vi "Periodic Tasks.vi"(8 "error in":errorcluster) -> ()   [LabVIEW 2018]
doc: "This VI runs in parallel to other robot code. It can contain as many user-defined periodic loops as you need. These can carry out PID or other sorts of timed response."
uses:
  <vilib>/Utility/config.llb/Read Key (String).vi
  Arm/Implementation/Arm Published Globals.vi
  <vilib>/Rock Robotics/Network Tables/NT Read String.vi
  <vilib>/Utility/config.llb/Write Key (String).vi
  Robot Global Data.vi
  <vilib>/Rock Robotics/SystemInterfaces/DIO/FPGA_DIOChannel.ctl
  <vilib>/ptbypt/NI_PtbyPt.lvlib
  <vilib>/Rock Robotics/WPI/ThirdParty/Phoenix-LabVIEW/Motor Controller/Controls/CTRE_Phoenix_MotorControl_MotionProfileTrajectoryPoint.ctl
  Arm/Arm Positions.ctl
  <vilib>/Utility/config.llb/NI_LVConfig.lvlib
  <vilib>/Rock Robotics/WPI/ThirdParty/Phoenix-LabVIEW/Pigeon IMU/CTRE_PigeonIMU_GetYPR.vi
  <vilib>/Rock Robotics/WPI/ThirdParty/Phoenix-LabVIEW/Motor Controller/Closed Loop/Motion Profile/CTRE_Phoenix_MotorControl_BufferedTrajectoryPointStream_WriteAll.vi
  <vilib>/Utility/file.llb/Read Delimited Spreadsheet (DBL).vi
  <vilib>/Rock Robotics/WPI/Switch/WPI_SwitchOpenCounting.vi
  <vilib>/Rock Robotics/WPI/Switch/WPI_SwitchOpenLimit.vi
panel:
  in  "Read FIle":bool
  out "Switch Pressed":bool
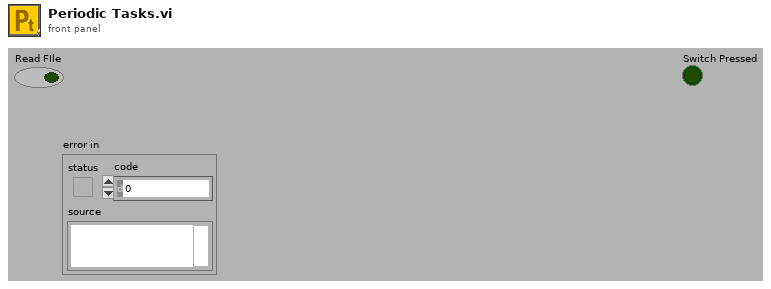
[diagram p1: front panel]
types:
  T1 = typedef "FPGA_DIOChannel.ctl" = enum8{"DIO 0", "DIO 1", "DIO 2", "DIO 3", "DIO 4", "DIO 5", "DIO 6", "DIO 7", "DIO 8", "DIO 9", "DIO MXP 0", "DIO MXP 1", "DIO MXP 2", "DIO MXP 3", "DIO MXP 4", "DIO MXP 5", "DIO MXP 6", "DIO MXP 7", "DIO MXP 8", "DIO MXP 9", "DIO MXP 10", "DIO MXP 11", "DIO MXP 12", "DIO MXP 13", "DIO MXP 14", "DIO MXP 15", "SPI Port CS1", "SPI Port CS2", "SPI Port CS3", "SPI Port MISO", "SPI Port MOSI", "Invalid"}
  T2 = typedef "WPI_JoystickDevRef.ctl" = cluster{"Device":T3}
  T3 = typedef "WPI_JoystickDeviceEnum.ctl" = enum16{"USB 0", "USB 1", "USB 2", "USB 3", "USB 4", "USB 5"}
  T4 = typedef "WPI_SwitchDevRef.ctl" = cluster{"DevStatus":errorcluster, "DIO Channel":T1, "CntIndex":T5, "Normally Closed":bool}
  T5 = typedef "FPGA_CounterCtrSystemIndex.ctl" = enum8{"Ctr 0", "Ctr 1", "Ctr 2", "Ctr 3", "Ctr 4", "Ctr 5", "Ctr 6", "Ctr 7", "Invalid"}
  T6 = typedef "CTRE_Phoenix_MotorControl_MotionProfileTrajectoryPoint.ctl" = cluster{"Position":dbl, "Velocity":dbl, "Arbitrary Feed Forward":dbl, "Auxiliary Position":dbl, "Auxiliary Velocity":dbl, "Auxiliary Arbitrary Feed Forward":dbl, "Profile Slot Select":i32, "Auxiliary Profile Slot Select":i32, "isLastPoint?":bool, "Zero Position?":bool, "durationMs":u32, "Use Aux PID?":bool}
  T7 = typedef "CTRE_Phoenix_MotorControl_BufferedTrajectoryPointStream_DeviceRef.ctl" = cluster{"Handle":u64, "Library Path":path}
  T8 = typedef "Arm Positions.ctl" = enum16{"Home Position", "Safe Position", "Hatch - Ground", "Hatch - Low", "Hatch - Middle", "Hatch - High", "Hatch - High 2", "Cargo - Low", "Cargo - Middle", "Cargo - High", "Cargo - Loading Station", "Hatch - Loading Station", "Cargo - Ground", "Turret - Left", "Turret - Front", "Turret - Right", "Turret - Back", "Climbing - Forward", "Hatch - Middle2"}
  T9 = typedef "CTRE_PigeonIMU_DeviceRef.ctl" = cluster{"DeviceStatus":errorcluster, "Device Number":u8, "Type":T10, "Device ID":u32, "Handle":u64, "UsageFrame":u32, "Library Path":path}
  T10 = typedef "CTRE_PigeonIMU_ConnectionType.ctl" = u32
  T11 = typedef "NI_LVConfig.lvlib/Config Data RefNum.ctl" = refnum<k1>
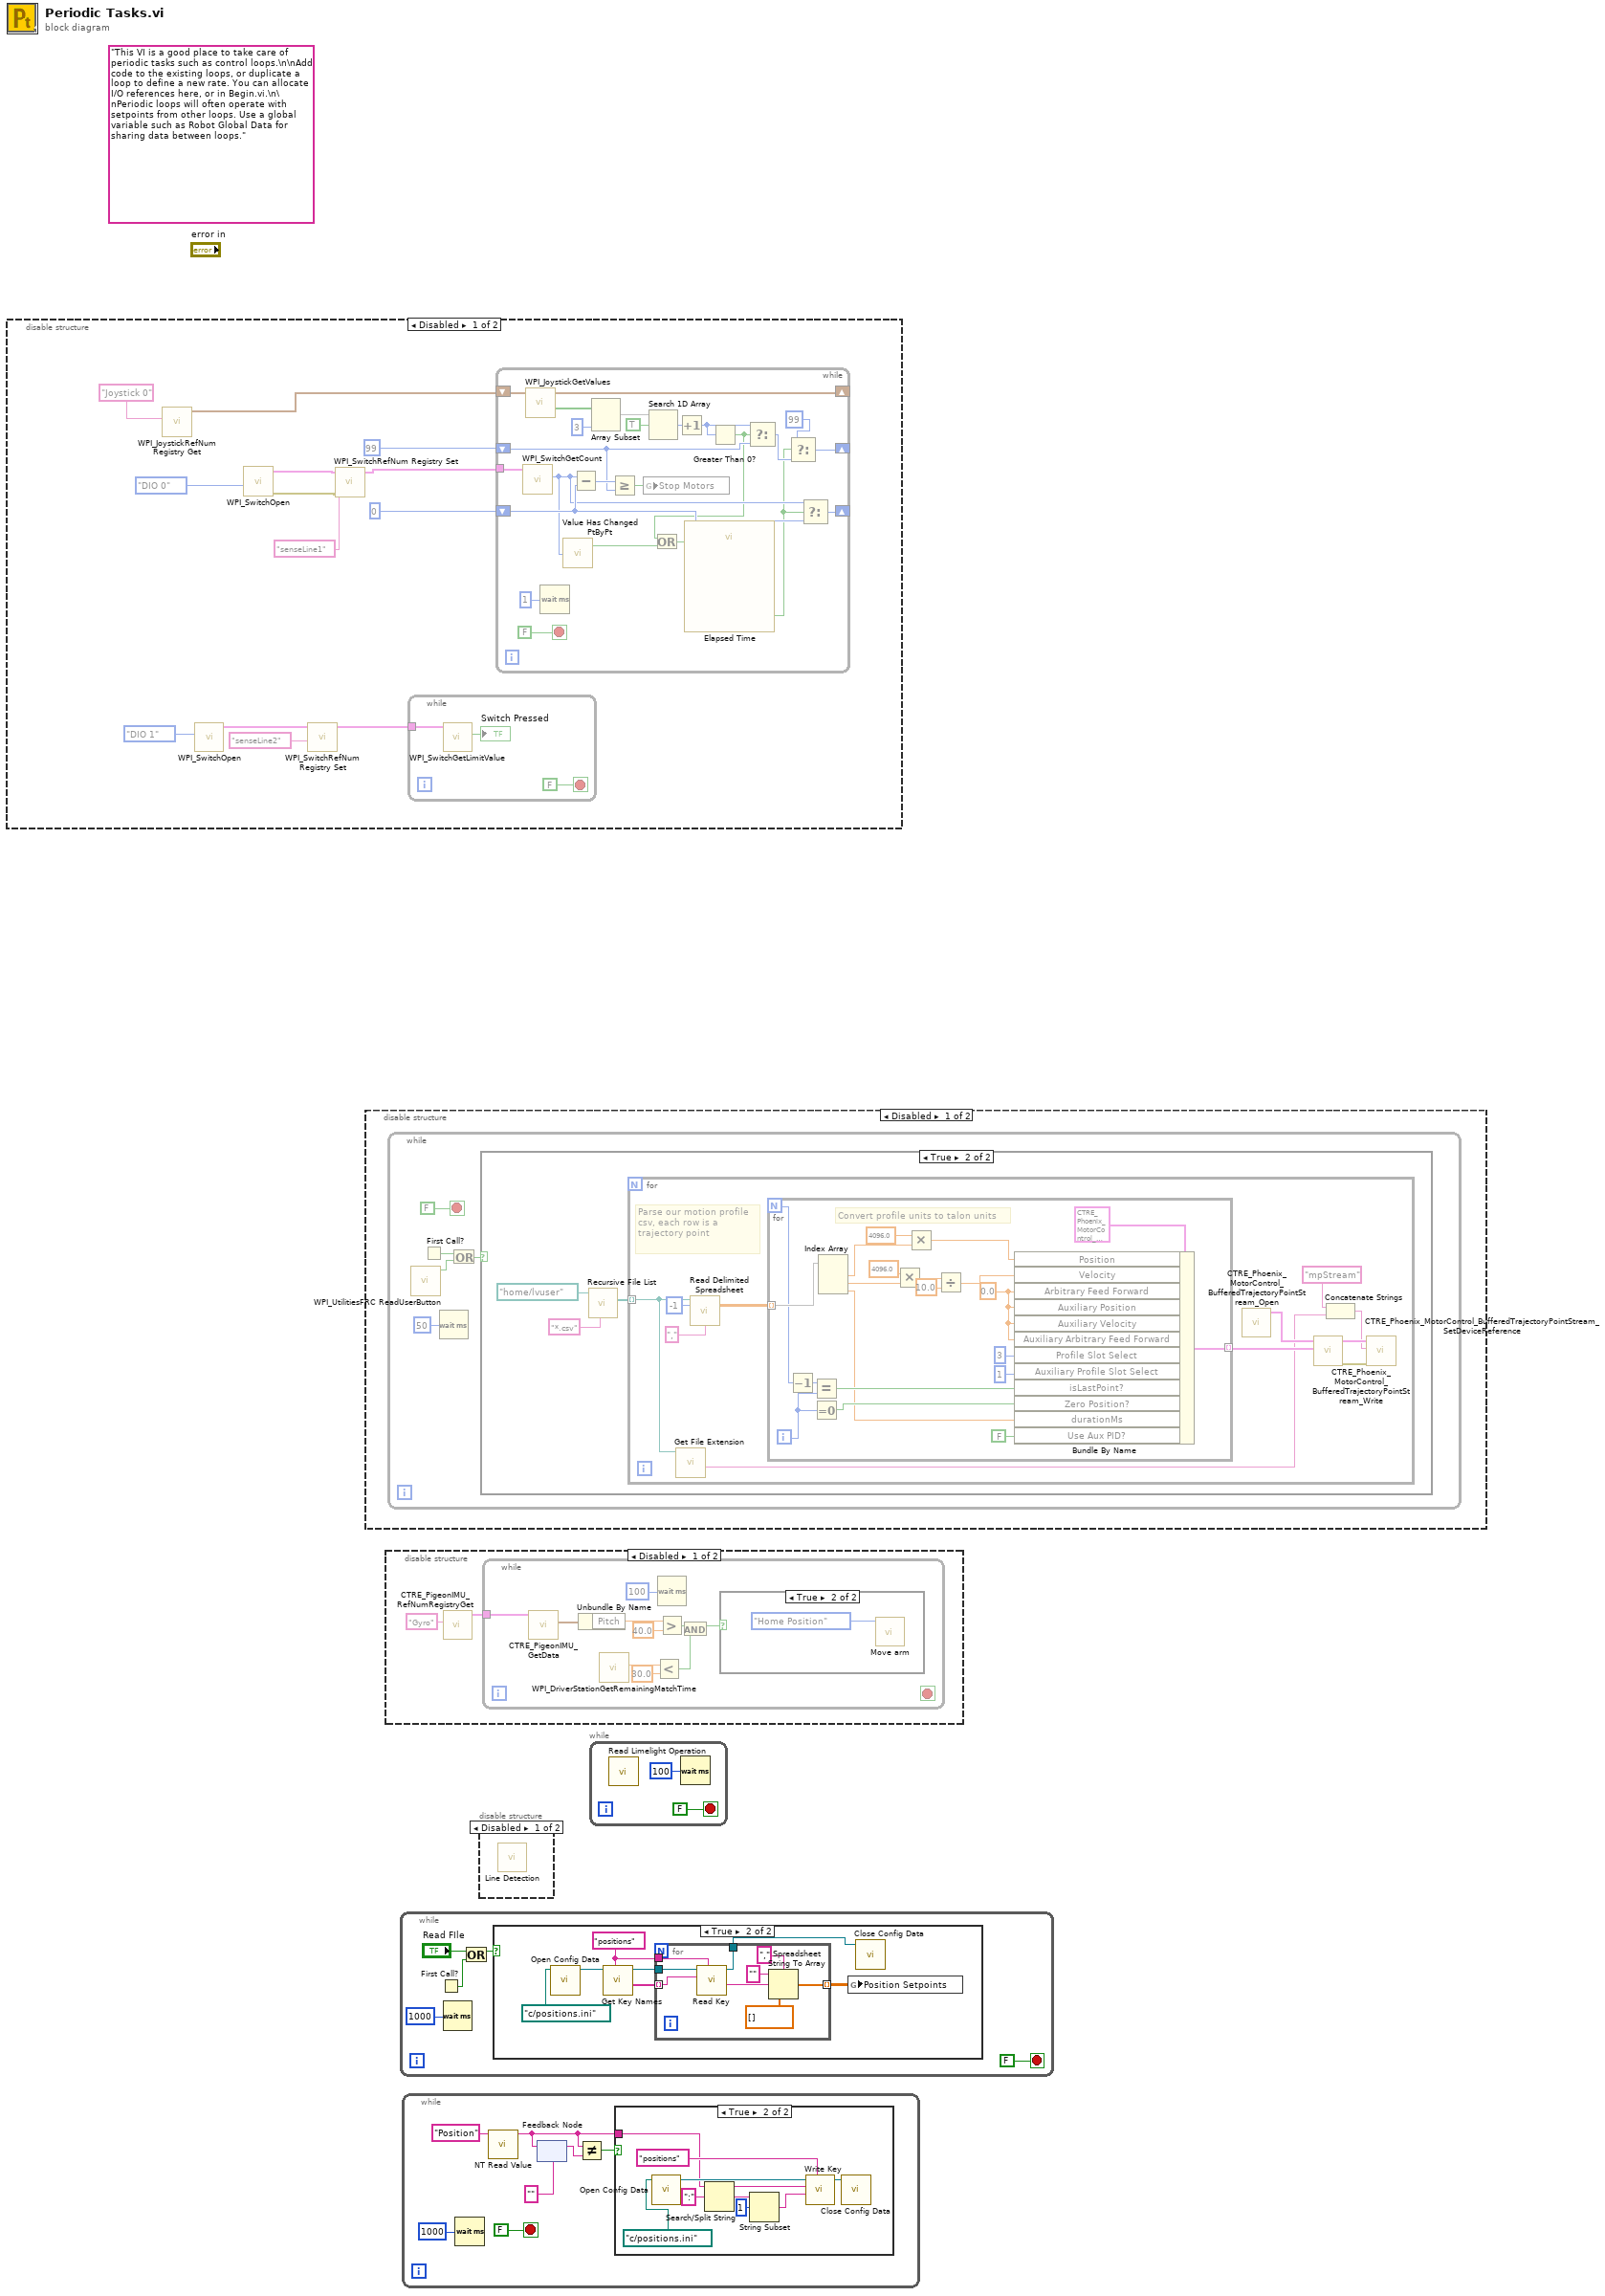
[diagram p0: block diagram]
diagram:
  (unwired) "This VI is a good place to take care of periodic tasks such as control loops.\n\nAdd code to the existing loops, or duplicate a loop to define a new rate. You can allocate I/O references here, or in Begin.vi.\n\nPeriodic loops will often operate with setpoints from other loops. Use a global variable such as Robot Global Data for sharing data between loops."
  n1 = disable-structure shown="Disabled" {
    frame Disabled {
      n2 = call <vilib>:"WPI_JoystickRefNum Registry Get.vi"("refnum name"="Joystick 0") -> ("JoystickDevRef"=w12:T2)  [unwired: 1 in, 9 out]
      n3 = call-poly <vilib>:"WPI_SwitchOpen.vi"("DIO Channel"=FPGA_DIOChannel."DIO 1") -> ("SwitchDevRef"=w3:T4)  [unwired: 9 in, 1 out]
      n4 = call-poly <vilib>:"WPI_SwitchOpen.vi"("DIO Channel"=FPGA_DIOChannel."DIO 0") -> ("error out"=w7:errorcluster, "SwitchDevRef"=w6:T4)  [unwired: 9 in]
      n5 = call <vilib>:"WPI_SwitchRefNum Registry Set.vi"("refnum name"="senseLine2", "SwitchDevRef"=w3) -> ("SwitchDevRef"=w2:T4)  [unwired: 8 in, 1 out]
      n6 = call <vilib>:"WPI_SwitchRefNum Registry Set.vi"("error in (no error)"=w7, "refnum name"="senseLine1", "SwitchDevRef"=w6) -> ("SwitchDevRef"=w5:T4)  [unwired: 7 in, 1 out]
      n7 = while {
        tunnel: w2 -> [w14]
        stop <- FALSE stop-if-true
        n8 = call <vilib>:"WPI_SwitchGetLimitValue.vi"("SwitchDevRef"=w14) -> ("Switch Pressed"=→"Switch Pressed":bool)  [unwired: 8 in, 2 out]
      }
      n9 = while {
        shift-right: [w37] -> _
        shift-left: w12 -> [w38]
        tunnel: w5 -> [w32]
        shift-right: [w30] -> _
        shift-left: 0 ("length") -> [w29]
        shift-right: [w22] -> _
        shift-left: 99 ("length") -> [w26]
        stop <- FALSE stop-if-true
        n10 = call <vilib>:"WPI_SwitchGetCount.vi"("SwitchDevRef"=w32) -> ("Switch Pressed Count"=w28:i32)  [unwired: 8 in, 2 out]
        n11 = call <vilib>:"WPI_JoystickGetValues.vi"("JoystickDevRef"=w38) -> ("Buttons"=w36:bool[], "JoystickDevRef"=w37:T2)  [unwired: 6 in, 3 out]
        n12 = Wait (ms)(milliseconds to wait=u32 1) -> ()  [unwired: 1 out]
        n13 = call <vilib>:"Value Has Changed PtByPt.vi"("input data point"=w28) -> ("has changed"=w19:bool)  [unwired: 1 in, 1 out]
        n14 = Subtract(x=w28, y=w29) -> (x-y=w27:i32)
        n15 = Array Subset(array=w36, length=3) -> (w34:bool[])  [unwired: 1 in]
        n16 = Greater Or Equal?(x=w27, y=w26) -> (x >= y?=w25:bool)
        n17 = global write "Robot Global Data.vi" "Stop Motors"(w25) -> ()
        n18 = Search 1D Array(1D array=w34, element=TRUE) -> (index of element=w31:i32)  [unwired: 1 in]
        n19 = Increment(x=w31) -> (x+1=w24:i32)
        n20 = Greater Than 0?(x=w24) -> (x > 0?=w17:bool)
        n21 = Or(x=w17, y=w19) -> (x .or. y?=w18:bool)
        n22 = call "Elapsed Time"("Reset"=w18) -> ("Time has Elapsed"=w21:bool)  [unwired: 11 in, 7 out]
        n23 = Select(t=w24, s=w17, f=w26) -> (s? t:f=w23:i32)
        n24 = Select(t=99 ("length"), s=w21, f=w23) -> (s? t:f=w22:i32)
        n25 = Select(t=w28, s=w21, f=w29) -> (s? t:f=w30:i32)
      }
    }
    frame Enabled {
    }
  }
  n26 = disable-structure shown="Disabled" {
    frame Disabled {
      n27 = while {
        stop <- FALSE stop-if-true
        n28 = call <vilib>:"WPI_UtilitiesFRC ReadUserButton.vi"() -> ("User Button"=w44:bool)  [unwired: 10 in, 1 out]
        n29 = First Call?() -> (First Call?: T/F=w45:bool)
        n30 = Wait (ms)(milliseconds to wait=u32 50) -> ()  [unwired: 1 out]
        n31 = Or(x=w45, y=w44) -> (x .or. y?=w42:bool)
        n32 = case shown="True" w42 {
          frame False {
          }
          frame True {
            n33 = call <vilib>:"Recursive File List.vi"("pattern"="*.csv", "Folder Path"=path "/home/lvuser" ("file path (use dialog)")) -> ("All Files in Dir"=w46:path[])  [unwired: 5 in, 4 out]
            n34 = for {
              tunnel: w46 -> [w50] mode=indexing
              # "Parse our motion profile csv, each row is a trajectory point"
              n35 = call <vilib>:"Get File Extension.vi"("file"=w50) -> ("filename without extension"=w49:string)  [unwired: 6 in, 4 out]
              n36 = call-poly <vilib>:"Read Delimited Spreadsheet.vi"("file path (dialog if empty)"=w50, "number of rows (all:-1)"=-1, "delimiter (\\t)"="," ("delimiter (\\t)")) -> ("all rows"=w55:dbl[][])  [unwired: 7 in, 5 out]
              n37 = for {
                N -> [w73]
                tunnel: w55 -> [w79] mode=indexing
                tunnel: [w69] -> w56 mode=indexing
                i -> [w72]
                w78 = 0.0 ("Arbitrary Feed Forward")
                # "Convert profile units to talon units"
                n38 = Decrement(x=w73) -> (x-1=w74:i32)
                n39 = Equal?(x=w74, y=w72) -> (x = y?=w75:bool)
                n40 = Equal To 0?(x=w72) -> (x = 0?=w71:bool)
                n41 = Index Array(array=w79) -> (element #1=w67:dbl, element #2=w61:dbl, element #3=w68:dbl)  [unwired: 3 in]
                n42 = Multiply(x=4096.0, y=w61) -> (x*y=w63:dbl)
                n43 = Multiply(x=4096.0, y=w67) -> (x*y=w65:dbl)
                n44 = Divide(x=w63, y=10.0) -> (x/y=w60:dbl)
                n45 = Bundle By Name(cluster=T6 {"Position"=0.0, "Velocity"=0.0, "Arbitrary Feed Forward"=0.0, "Auxiliary Position"=0.0, "Auxiliary Velocity"=0.0, "Auxiliary Arbitrary Feed Forward"=0.0, "Profile Slot Select"=0, "Auxiliary Profile Slot Select"=0, "isLastPoint?"=FALSE, "Zero Position?"=FALSE, "durationMs"=0, "Use Aux PID?"=FALSE} ("Trajectory Point"), "Position"=w65, "Velocity"=w60, "Arbitrary Feed Forward"=w78, "Auxiliary Position"=w78, "Auxiliary Velocity"=w78, "Auxiliary Arbitrary Feed Forward"=w78, "Profile Slot Select"=3, "Auxiliary Profile Slot Select"=1, "isLastPoint?"=w75, "Zero Position?"=w71, "durationMs"=w68, "Use Aux PID?"=FALSE) -> (w69:T6)
              }
              n46 = call <vilib>:"CTRE_Phoenix_MotorControl_BufferedTrajectoryPointStream_Open.vi"() -> ("BufferedTrajectoryPointStream_DevRef"=w57:T7)  [unwired: 10 in, 1 out]
              n47 = call-poly <vilib>:"CTRE_Phoenix_MotorControl_BufferedTrajectoryPointStream_Write.vi"("Motion Profile Trajectory Point Array"=w56, "BufferedTrajectoryPointStream_DevRef"=w57) -> ("error out"=w59:errorcluster, "BufferedTrajectoryPointStream_DevRef"=w58:T7)  [unwired: 8 in]
              n48 = Concatenate Strings("mpStream" ("refnum name"), w49) -> (w52:string)
              n49 = call <vilib>:"CTRE_Phoenix_MotorControl_BufferedTrajectoryPointStream_SetDeviceReference.vi"("error in (no error)"=w59, "refnum name"=w52, "BufferedTrajectoryPointStream_DevRef"=w58) -> ()  [unwired: 7 in, 2 out]
            }
          }
        }
      }
    }
    frame Enabled {
    }
  }
  n50 = disable-structure shown="Disabled" {
    frame Disabled {
      n51 = call <vilib>:"CTRE_PigeonIMU_RefNumRegistryGet.vi"("refnum name"="Gyro") -> ("PigeonIMUDevRef"=w81:T9)  [unwired: 9 in, 1 out]
      n52 = while {
        tunnel: w81 -> [w91]
        stop <- _ stop-if-true
        n53 = call-poly <vilib>:"CTRE_PigeonIMU_GetData.vi"("PigeonIMUDevRef"=w91) -> ("Yaw Pitch Roll"=w92:cluster{"Yaw":dbl, "Pitch":dbl, "Roll":dbl})  [unwired: 8 in, 2 out]
        n54 = Unbundle By Name(w92) -> ("Pitch"=w90:dbl)
        n55 = call <vilib>:"WPI_DriverStationGetRemainingMatchTime.vi"() -> ("Match Time(s)"=w84:sgl)  [unwired: 10 in, 1 out]
        n56 = Less?(x=w84, y=sgl 30.0) -> (x < y?=w85:bool)
        n57 = Wait (ms)(milliseconds to wait=u32 100) -> ()  [unwired: 1 out]
        n58 = Greater?(x=w90, y=40.0) -> (0:w89:bool)
        n59 = And(x=w89, y=w85) -> (x .and. y?=w86:bool)
        n60 = case shown="True" w86 {
          frame False {
          }
          frame True {
            n61 = call "Move arm.vi"("Arm Position"=Arm_Positions."Home Position") -> ()  [unwired: 10 in, 1 out]
          }
        }
      }
    }
    frame Enabled {
    }
  }
  n62 = while {
    stop <- FALSE stop-if-true
    n63 = First Call?() -> (First Call?: T/F=w95:bool)
    n64 = Wait (ms)(milliseconds to wait=u32 1000) -> ()  [unwired: 1 out]
    n65 = Or(x="Read FIle", y=w95) -> (x .or. y?=w96:bool)
    n66 = case shown="True" w96 {
      frame False {
      }
      frame True {
        w103 = "positions" ("section")
        n67 = call <vilib>:"Open Config Data.vi"("configuration file path"=path "c:/positions.ini") -> ("refnum"=w100:T11)  [unwired: 8 in, 2 out]
        n68 = call <vilib>:"Get Key Names.vi"("section"=w103, "refnum"=w100) -> ("key names"=w102:string[], "refnum out"=w105:T11)  [unwired: 6 in, 2 out]
        n69 = for {
          tunnel: w105 -> [w114]
          tunnel: [w111] -> w104 mode=indexing
          tunnel: w103 -> [w108]
          tunnel: w102 -> [w107] mode=indexing
          tunnel: [w106] -> w99
          n70 = call-poly <vilib>:"Read Key.vi"("section"=w108, "key"=w107, "refnum"=w114) -> ("value"=w112:string, "refnum out"=w106:T11)  [unwired: 5 in, 2 out]
          n71 = Spreadsheet String To Array(delimiter (Tab)=",", format string="", spreadsheet string=w112, array type (2D Dbl)=dbl[] []) -> (array=w111:dbl[])
        }
        n72 = global write "Arm Published Globals.vi" "Position Setpoints"(w104) -> ()
        n73 = call <vilib>:"Close Config Data.vi"("refnum"=w99) -> ()  [unwired: 9 in, 2 out]
      }
    }
  }
  n74 = while {
    stop <- FALSE stop-if-true
    n75 = Wait (ms)(milliseconds to wait=u32 1000) -> ()  [unwired: 1 out]
    n76 = call-poly <vilib>:"NT Read Value.vi"("Name"="Position") -> ("String"=w116:string)  [unwired: 9 in, 1 out]
    n77 = feedback-in #1(w116) -> ()
    n78 = feedback #1("" ("String")) -> (w117:string)
    n79 = Not Equal?(x=w116, y=w117) -> (x != y?=w115:bool)
    n80 = case shown="True" w115 {
      tunnel: w116 -> [_ w126]
      frame False {
      }
      frame True {
        n81 = call <vilib>:"Open Config Data.vi"("configuration file path"=path "c:/positions.ini") -> ("refnum"=w130:T11)  [unwired: 8 in, 2 out]
        n82 = Search/Split String(string=w126, search string/char (-)=":") -> (substring before match=w127:string, match + rest of string=w124:string)  [unwired: 1 in, 1 out]
        n83 = String Subset(string=w124, offset (0)=1) -> (substring=w122:string)  [unwired: 1 in]
        n84 = call-poly <vilib>:"Write Key.vi"("section"="positions", "value"=w122, "key"=w127, "refnum"=w130) -> ("refnum out"=w128:T11)  [unwired: 5 in, 2 out]
        n85 = call <vilib>:"Close Config Data.vi"("refnum"=w128) -> ()  [unwired: 9 in, 2 out]
      }
    }
  }
  n86 = disable-structure shown="Disabled" {
    frame Disabled {
      n87 = call "Line Detection.vi"() -> ()  [unwired: 12 in]
    }
    frame Enabled {
    }
  }
  n88 = while {
    stop <- FALSE stop-if-true
    n89 = call "Read Limelight Operation.vi"() -> ()  [unwired: 9 in, 3 out]
    n90 = Wait (ms)(milliseconds to wait=u32 100) -> ()  [unwired: 1 out]
  }
